vi "Show Mission Screen.vi"(8 "error in":errorcluster, 11 "Base Software in":refnum<class "Main.lvclass">) -> (0 "error out":errorcluster, 3 "Base Software out":refnum<class "Main.lvclass">)   [LabVIEW 2023, in "Main.lvlib" / "Main.lvclass"]
uses:
  Project/Main.lvclass
  C:/Users/Public/Documents/Development/builds/Engine/Engine.lvlibp/Project/Engine.lvclass
  Project/Main.lvclass/Main.ctl
  builds/Engine/Engine.lvlibp/Accessors/Read Directory.vi
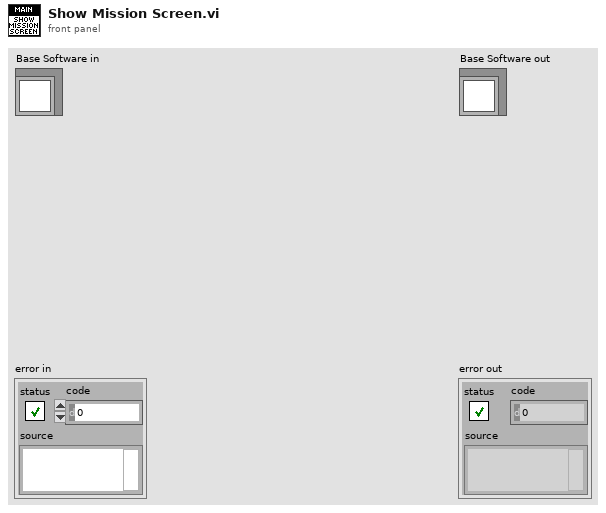
[diagram p1: front panel]
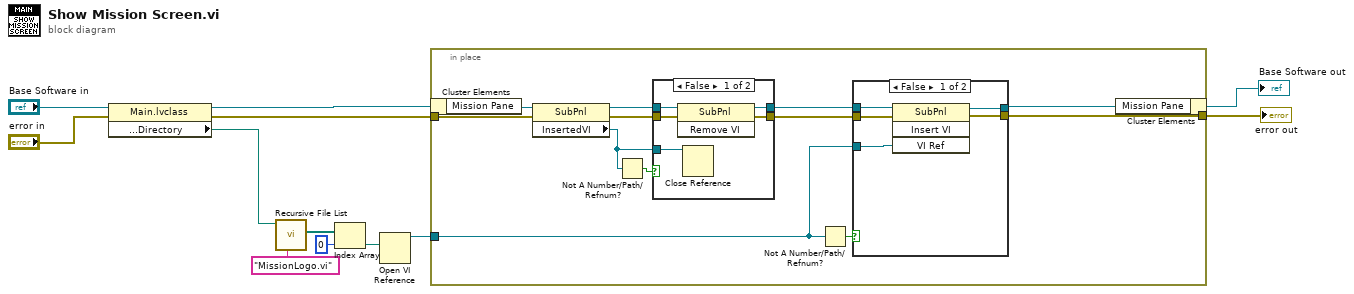
[diagram p0: block diagram]
diagram:
  n1 = property class="Main.lvclass"(reference="Base Software in", error in="error in") -> (reference out=w6:refnum<class "Main.lvclass">, error out=w2:errorcluster, "Accessors:Application:Information:Directory"=w11:path)
  n2 = call <vilib>:"Recursive File List.vi"("pattern"="MissionLogo.vi" ("name or relative path"), "Folder Path"=w11) -> ("All Files in Dir"=w9:path[])  [unwired: 5 in, 4 out]
  n3 = Index Array(array=w9, index=0) -> (element=w8:path)
  n4 = Open VI Reference(vi path=w8) -> (vi reference=w4:refnum<vi>)  [unwired: 5 in, 1 out]
  n5 = in-place {
    in-place-border: w4 -> [w15]
    in-place-border: w2 -> [w14]
    in-place-border: [w13] -> w1
    n6 = in-place-cluster #1(w6) -> ("Mission Pane"=w17:refnum<vi>)
    n7 = property class="SubPnl"(reference=w17, error in=w14) -> (reference out=w20:refnum<vi>, error out=w21:errorcluster, "InsertedVI"=w23:refnum<vi>)
    n8 = Not A Number/Path/Refnum?(number/path/refnum=w23) -> (NaN/Path/Refnum?=w22:bool)
    n9 = case shown="False" w22 {
      tunnel: [w29 w31] -> w18
      tunnel: [w28 w30] -> w24
      tunnel: w20 -> [w27 w31]
      tunnel: w21 -> [w26 w30]
      tunnel: w23 -> [w25 _]
      frame False {
        n10 = invoke class="SubPnl" method="Remove VI"(reference=w27, error in=w26) -> (reference out=w29:refnum<vi>, error out=w28:errorcluster)  [unwired: 1 in, 1 out]
        n11 = Close Reference(reference=w25) -> ()  [unwired: 1 in, 1 out]
      }
      frame True {
      }
    }
    n12 = Not A Number/Path/Refnum?(number/path/refnum=w15) -> (NaN/Path/Refnum?=w19:bool)
    n13 = case shown="False" w19 {
      tunnel: [w36 w38] -> w16
      tunnel: w18 -> [w35 w38]
      tunnel: w24 -> [w34 w37]
      tunnel: [w33 w37] -> w13
      tunnel: w15 -> [w32 _]
      frame False {
        n14 = invoke class="SubPnl" method="Insert VI"(reference=w35, error in=w34, "VI Ref"=w32) -> (reference out=w36:refnum<vi>, error out=w33:errorcluster)  [unwired: 1 in, 2 out]
      }
      frame True {
      }
    }
    n15 = in-place-cluster #1("Mission Pane"=w16) -> (→"Base Software out":refnum<class "Main.lvclass">)
  }
  "error out" <- w1
